vi "Deposit fgv.vi"(7 "Command":enum16{"Set User Input", "Get User Input"}(ring), 8 "error in (no error)":errorcluster, 10 "User Input IN  in":string) -> (0 "error out":errorcluster, 2 "User Input IN  out":string)   [LabVIEW 2013]
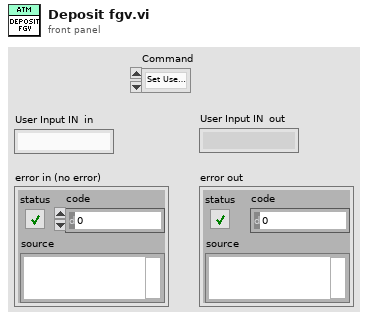
[diagram p1: front panel]
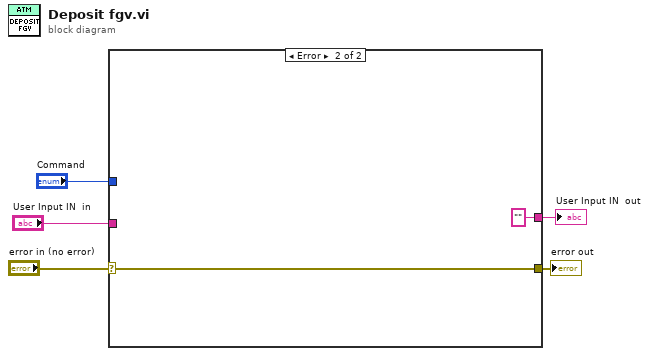
[diagram p0: block diagram]
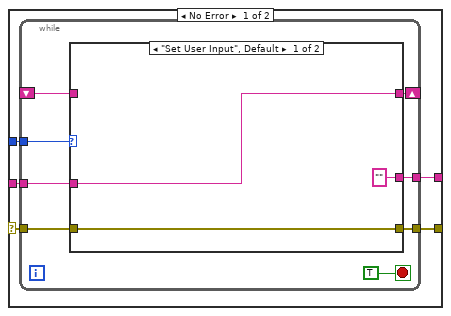
[diagram p2: hidden frame]
diagram:
  n1 = case shown="Error" "error in (no error)" {
    selector: "error in (no error)" -> [w7 w25]
    tunnel: "Command" -> [w10 _]
    tunnel: "User Input IN  in" -> [w9 _]
    tunnel: [w8 "" ("User Input IN  in")] -> w3
    tunnel: [w6 w25] -> w1
    frame No Error {
      n2 = while {
        tunnel: w10 -> [w17]
        tunnel: w9 -> [w16]
        shift-right: [w15] -> _
        shift-left: _ -> [w14]
        tunnel: [w13] -> w8
        tunnel: w7 -> [w12]
        tunnel: [w11] -> w6
        stop <- TRUE stop-if-true
        n3 = case shown="\"Set User Input\", Default" w17 {
          tunnel: w16 -> [w21 _]
          tunnel: [w21 w23] -> w15
          tunnel: w14 -> [_ w23]
          tunnel: ["" ("User Input IN  in") w23] -> w13
          tunnel: w12 -> [w20 w22]
          tunnel: [w20 w22] -> w11
          frame "Set User Input", Default {
          }
          frame "Get User Input" {
          }
        }
      }
    }
    frame Error {
    }
  }
  "User Input IN  out" <- w3
  "error out" <- w1
